vi "rfStore.vi"(6 "channel_name":string, 8 "error in (no error)":errorcluster, 9 "rf.lvclass":refnum<class "rf.lvclass">, 10 "action":enum16{"Write", "Read", "Reset"}(ring), 11 "rfArray in":refnum<class "rfArray.lvclass">) -> (0 "error out":errorcluster, 1 "rf out":refnum<class "rf.lvclass">, 2 "found?":bool, 3 "rfArray out":refnum<class "rfArray.lvclass">)   [LabVIEW 2009, in "Tools.lvlib" / "Scripting.lvlib" / "rfArray.lvclass"]
uses:
  rfArray.lvclass
  Rf Event/rf.lvclass
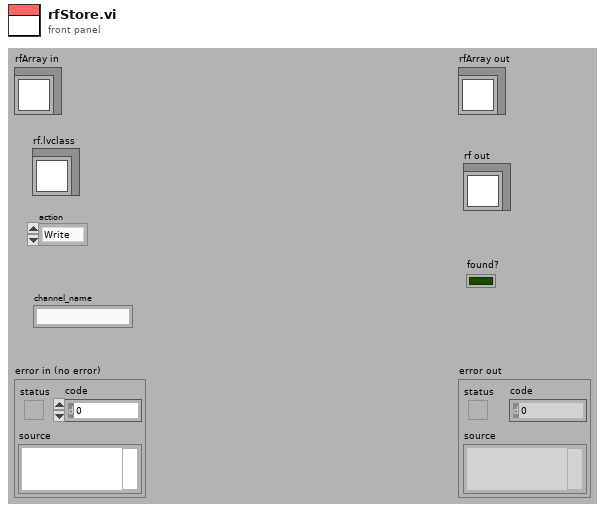
[diagram p1: front panel]
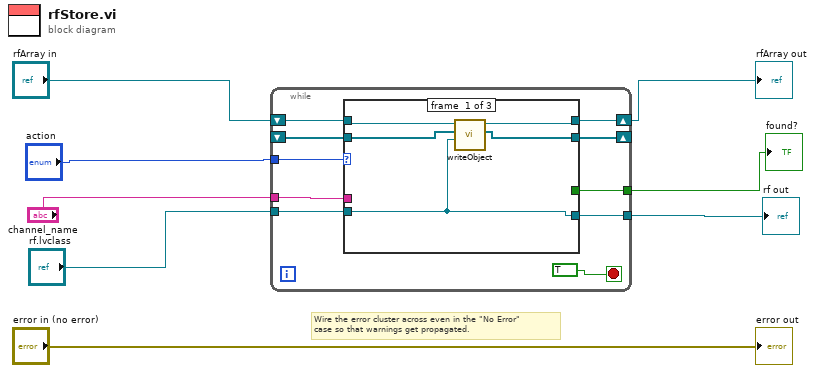
[diagram p0: block diagram]
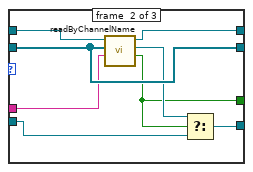
[diagram p2: hidden frame]
diagram:
  # "Wire the error cluster across even in the \"No Error\"\ncase so that warnings get propagated."
  n1 = while {
    tunnel: "action" -> [w17]
    shift-right: [w14] -> _
    shift-left: _ -> [w16]
    tunnel: "rf.lvclass" -> [w15]
    shift-right: [w12] -> w4
    shift-left: "rfArray in" -> [w13]
    tunnel: [w11] -> w2
    tunnel: "channel_name" -> [w10]
    tunnel: [w9] -> w1
    stop <- TRUE stop-if-true
    n2 = case shown="\"Reset\"" w17 {
      tunnel: w16 -> [w21 w29 _]
      tunnel: w15 -> [w19 w26 _]
      tunnel: [w20 w29 _] -> w14
      tunnel: w13 -> [w23 w31 w32]
      tunnel: [w22 w30 w32] -> w12
      tunnel: [w19 w25 _] -> w11
      tunnel: w10 -> [_ w28 _]
      tunnel: [_ w24 _] -> w9
      frame #0 {
        n3 = call "writeObject.vi"("rf.lvclass"=w19, "Array"=w21, "rfArray in"=w23) -> ("Array out"=w20:refnum<class "rf.lvclass">[], "rfArray out"=w22:refnum<class "rfArray.lvclass">)  [unwired: 6 in, 1 out]
      }
      frame #1 {
        n4 = call "readByChannelName.vi"("channel_name"=w28, "Array"=w29, "rfArray in"=w31) -> ("found?"=w24:bool, "rf.lvclass"=w27:refnum<class "rf.lvclass">, "rfArray out"=w30:refnum<class "rfArray.lvclass">)  [unwired: 5 in, 1 out]
        n5 = Select(t=w27, s=w24, f=w26) -> (s? t:f=w25:refnum<class "rf.lvclass">)
      }
      frame #2 {
      }
    }
  }
  "rfArray out" <- w4
  "rf out" <- w2
  "found?" <- w1
  "error out" <- "error in (no error)"
